vi "Stick Angle.vi"(10 "X":dbl, 11 "Y":dbl) -> (0 "Stick Pressed":bool, 3 "Angle":dbl)   [LabVIEW 2013]
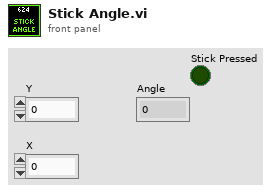
[diagram p1: front panel]
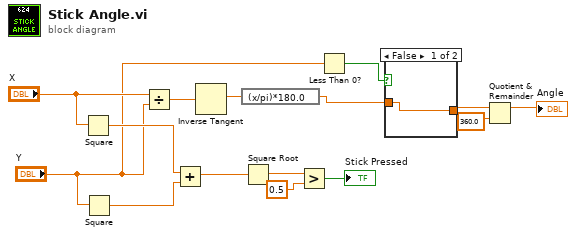
[diagram p0: block diagram]
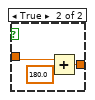
[diagram p2: hidden frame]
diagram:
  n1 = Square(x="X") -> (x^2=w13:dbl)
  n2 = Square(x="Y") -> (x^2=w12:dbl)
  n3 = Divide(x="X", y="Y") -> (x/y=w14:dbl)
  n4 = Add(x=w13, y=w12) -> (x+y=w11:dbl)
  n5 = Inverse Tangent(1:w14) -> (0:w15:dbl)
  n6 = expression code="(x/pi)*180.0" ("radians to degrees")(w15) -> (w5:dbl)
  n7 = Square Root(x=w11) -> (sqrt(x)=w10:dbl)
  n8 = Greater?(x=w10, y=0.5) -> (0:→"Stick Pressed":bool)
  n9 = Less Than 0?(x="Y") -> (x < 0?=w4:bool)
  n10 = case shown="False" w4 {
    tunnel: w5 -> [w16 w19]
    tunnel: [w16 w17] -> w3
    frame False {
    }
    frame True {
      n11 = Add(x=w19, y=180.0) -> (x+y=w17:dbl)
    }
  }
  n12 = Quotient & Remainder(x=w3, y=360.0) -> (x-y*floor(x/y)=→"Angle":dbl)  [unwired: 1 out]
